vi "New.vi"(8 "error in (no error)":errorcluster, 11 "menu refnum":refnum<vi>) -> (0 "error out":errorcluster, 3 "menu out":refnum<class "menu.lvclass">)   [LabVIEW 2009, in "menu.lvclass"]
uses:
  menu.lvclass
  menu.lvclass/menu.ctl
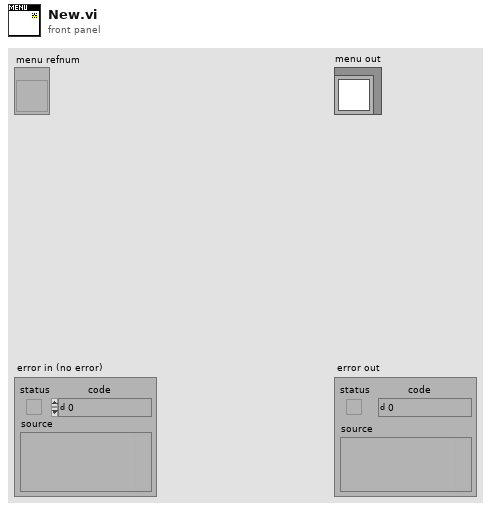
[diagram p1: front panel]
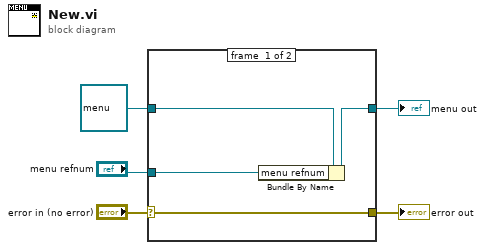
[diagram p0: block diagram]
diagram:
  n1 = case shown="No Error" "error in (no error)" {
    selector: "error in (no error)" -> [w8 w11]
    tunnel: [w8 w11] -> w2
    tunnel: [w7 w10] -> w4
    tunnel: refnum<class "menu.lvclass"> refnum ("menu in") -> [w9 w10]
    tunnel: "menu refnum" -> [w6 _]
    frame #0 {
      n2 = Bundle By Name(cluster=w9, "menu refnum"=w6) -> (w7:refnum<class "menu.lvclass">)
    }
    frame #1 {
    }
  }
  "menu out" <- w4
  "error out" <- w2
